vi "RDAOutcouterByMachine.vi"(7 "Machine":string="QAMT08", 8 "error in (no error) 2":errorcluster, 9 "report in":refnum<class "NI_report.lvclass">, 10 "error in (no error)":errorcluster, 11 "connection reference":T1) -> (0 "error in (no error) 3":errorcluster, 1 "report in 2":refnum<class "NI_report.lvclass">, 2 "error out":errorcluster, 3 "connection reference 2":T1)   [LabVIEW 2012]
uses:
  <vilib>/addons/database/Connection.llb/Conn ObjectReference.ctl
  <vilib>/Utility/NIReport.llb/NI_report.lvclass
  <vilib>/addons/database/Auxilliary.llb/DB Tools Cursor Type.ctl
  <vilib>/addons/database/Connection.llb/Conn Execute.vi
  <vilib>/addons/database/Recordset.llb/Rec Fetch Recordset Data (R).vi
  <vilib>/addons/database/Recordset.llb/Rec Destroy - Connection.vi
  <vilib>/addons/database/_DB Variant To Data/Database Variant To Data.xnode
  <vilib>/Utility/NIReport.llb/Excel/NI_Excel.lvclass
  <vilib>/addons/database/NI_Database_API.lvlib
panel:
  out "concatenated string":string
  in  "?":cluster{"start row":i32, "start column":i32}
  in  "?":cluster{"start row":i32, "start column":i32}
  in  "?":cluster{"start row":i32, "start column":i32}
  in  "?":cluster{"start row":i32, "start column":i32}
  in  "?":cluster{"start row":i32, "start column":i32}
  in  "?":cluster{"start row":i32, "start column":i32}
  in  "?":cluster{"start row":i32, "start column":i32}
  in  "?":cluster{"start row":i32, "start column":i32}
  in  "?":cluster{"start row":i32, "start column":i32}
  in  "?":cluster{"start row":i32, "start column":i32}
  in  "?":cluster{"start row":i32, "start column":i32}
  in  "?":cluster{"start row":i32, "start column":i32}
  in  "?":cluster{"start row":i32, "start column":i32}
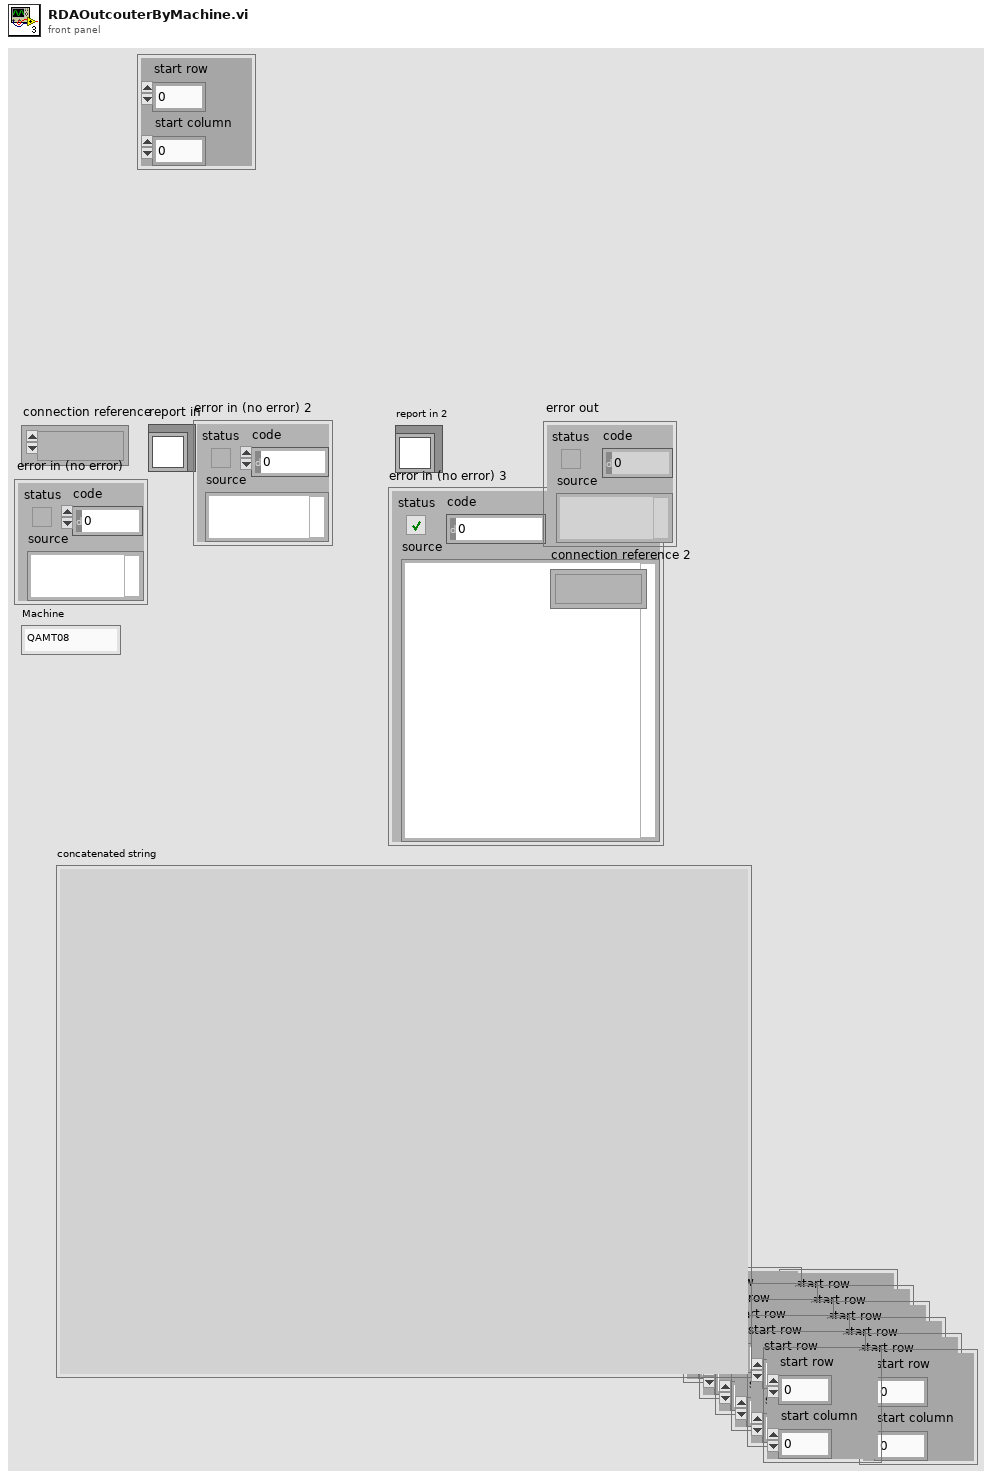
[diagram p1: front panel]
types:
  T1 = typedef "NI_Database_API.lvlib/Conn ObjectReference.ctl" = refnum<k1>
  T2 = typedef "NI_Database_API.lvlib/DB Tools Cursor Type.ctl" = enum16{"forward-only", "keyset", "dynamic", "static"}
  T3 = typedef "NI_Database_API.lvlib/Rec ObjectReference.ctl" = refnum<k1>
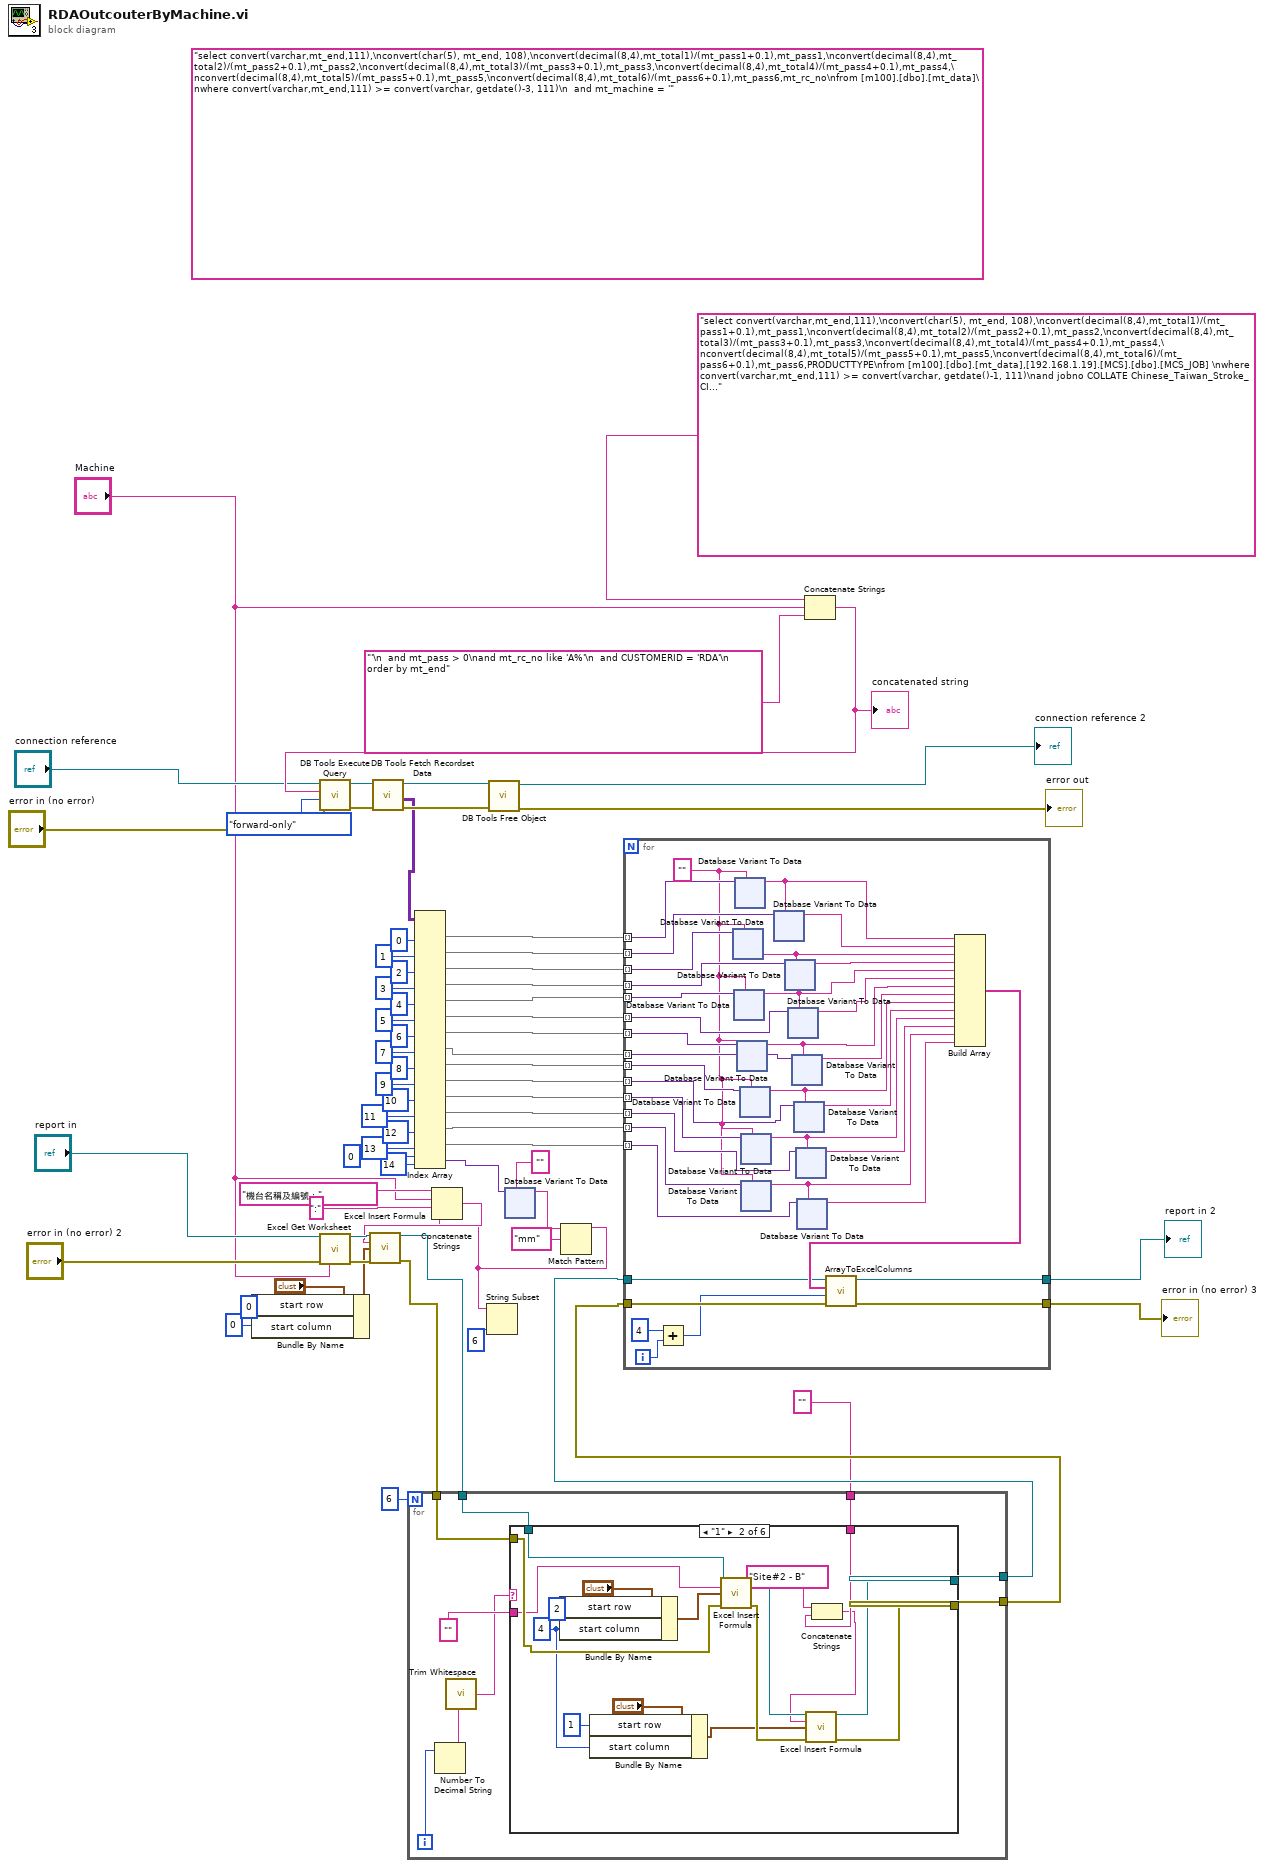
[diagram p0: block diagram]
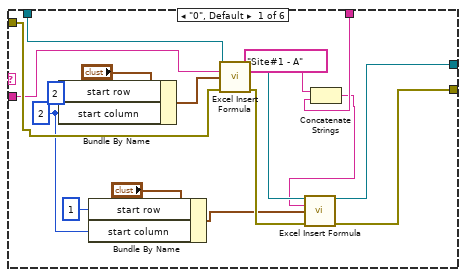
[diagram p2: hidden frame]
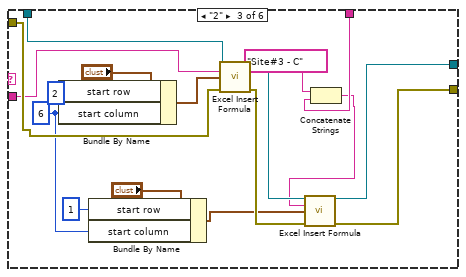
[diagram p3: hidden frame]
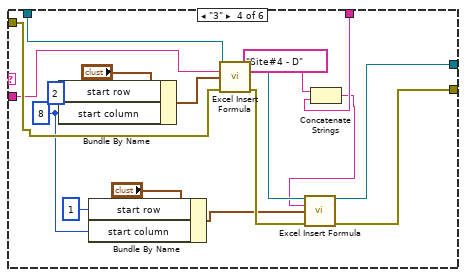
[diagram p4: hidden frame]
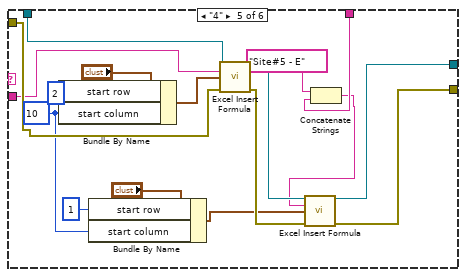
[diagram p5: hidden frame]
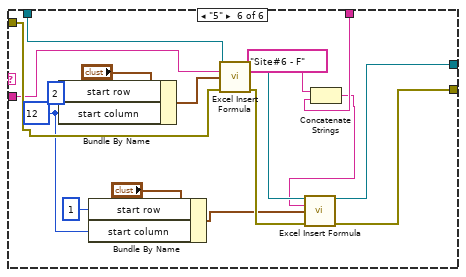
[diagram p6: hidden frame]
diagram:
  (unwired) "select convert(varchar,mt_end,111),\nconvert(char(5), mt_end, 108),\nconvert(decimal(8,4),mt_total1)/(mt_pass1+0.1),mt_pass1,\nconvert(decimal(8,4),mt_total2)/(mt_pass2+0.1),mt_pass2,\nconvert(decimal(8,4),mt_total3)/(mt_pass3+0.1),mt_pass3,\nconvert(decimal(8,4),mt_total4)/(mt_pass4+0.1),mt_pass4,\nconvert(decimal(8,4),mt_total5)/(mt_pass5+0.1),mt_pass5,\nconvert(decimal(8,4),mt_total6)/(mt_pass6+0.1),mt_pass6,mt_rc_no\nfrom [m100].[dbo].[mt_data]\nwhere convert(varchar,mt_end,111) >= convert(varchar, getdate()-3, 111)\n  and mt_machine = '" ("SQL query")
  n1 = Bundle By Name(cluster="?", "start row"=0, "start column"=0) -> (w28:cluster{"start row":i32, "start column":i32})
  n2 = call <vilib>:"Excel Get Worksheet.vi"("report in"="report in", "error in (no error)"="error in (no error) 2", "name (\"\")"="Machine") -> ("report out"=w33:refnum<class "NI_report.lvclass">, "error out"=w32:errorcluster)  [unwired: 11 in]
  n3 = Concatenate Strings("select convert(varchar,mt_end,111),\nconvert(char(5), mt_end, 108),\nconvert(decimal(8,4),mt_total1)/(mt_pass1+0.1),mt_pass1,\nconvert(decimal(8,4),mt_total2)/(mt_pass2+0.1),mt_pass2,\nconvert(decimal(8,4),mt_total3)/(mt_pass3+0.1),mt_pass3,\nconvert(decimal(8,4),mt_total4)/(mt_pass4+0.1),mt_pass4,\nconvert(decimal(8,4),mt_total5)/(mt_pass5+0.1),mt_pass5,\nconvert(decimal(8,4),mt_total6)/(mt_pass6+0.1),mt_pass6,PRODUCTTYPE\nfrom [m100].[dbo].[mt_data],[192.168.1.19].[MCS].[dbo].[MCS_JOB] \nwhere convert(varchar,mt_end,111) >= convert(varchar, getdate()-1, 111)\nand jobno COLLATE Chinese_Taiwan_Stroke_CI_AS = mt_rc_no\n  and mt_machine = '" ("string"), "Machine", "'\n  and mt_pass > 0\nand mt_rc_no like 'A%'\n  and CUSTOMERID = 'RDA'\n  order by mt_end" ("SQL query")) -> (w34:string)
  "concatenated string" <- w34
  n4 = call-poly <vilib>:"DB Tools Execute Query.vi"("error in (no error)"="error in (no error)", "cursor type"=DB_Tools_Cursor_Type."forward-only", "SQL query"=w34, "connection reference"="connection reference") -> ("error out"=w69:errorcluster, "recordset reference"=w68:T3)  [unwired: 4 in]
  n5 = call-poly <vilib>:"DB Tools Fetch Recordset Data.vi"("error in (no error)"=w69, "recordset reference"=w68) -> ("error out"=w66:errorcluster, "recordset data"=w64:variant[][], "recordset reference out"=w67:T3)  [unwired: 3 in]
  n6 = Index Array(array=w64, index (col) #1=0 ("disabled index (col)"), index (col) #2=1 ("index (col)"), index (col) #3=2 ("index (col)"), index (col) #4=3 ("index (col)"), index (col) #5=4 ("index (col)"), index (col) #6=5 ("index (col)"), index (col) #7=6 ("index (col)"), index (col) #8=7 ("index (col)"), index (col) #9=8 ("index (col)"), index (col) #10=9 ("index (col)"), index (col) #11=10 ("index (col)"), index (col) #12=11 ("index (col)"), index (col) #13=12 ("index (col)"), index (col) #14=13 ("index (col)"), index (row) #15=0 ("disabled index (row)"), index (col) #15=14 ("disabled index (col)")) -> (element #1=w61:variant[], element #2=w60:variant[], element #3=w59:variant[], element #4=w48:variant[], element #5=w47:variant[], element #6=w46:variant[], element #7=w45:variant[], element #8=w44:variant[], element #9=w43:variant[], element #10=w42:variant[], element #11=w41:variant[], element #12=w40:variant[], element #13=w37:variant[], element #14=w36:variant[], element #15=w14:variant)  [unwired: 14 in]
  n7 = call-poly <vilib>:"DB Tools Free Object.vi"("error in (no error)"=w66, "recordset reference"=w67) -> ("error out"=→"error out":errorcluster, "connection reference"=→"connection reference 2":T1)  [unwired: 8 in]
  n8 = xnode "Database Variant To Data"("database variant"=w14, "type"="") -> ("data"=w12:string)  [unwired: 1 in, 1 out]
  n9 = Match Pattern(string=w12, regular expression="mm") -> (before substring=w4:string)  [unwired: 1 in, 3 out]
  n10 = Concatenate Strings("機台名稱及編號：" ("formula"), "Machine", ":" ("string"), w4) -> (w27:string)
  n11 = call <vilib>:"Excel Insert Formula.vi"("report in"=w33, "formula"=w27, "start (0, 0)"=w28, "error in (no error)"=w32) -> ("report out"=w10:refnum<class "NI_report.lvclass">, "error out"=w9:errorcluster)  [unwired: 10 in]
  n12 = for {
    N: 6 -> [_]
    tunnel: w10 -> [w78]
    tunnel: w9 -> [w77]
    tunnel: [w76] -> w8
    tunnel: [w75] -> w7
    tunnel: "" -> [w74]
    i -> [w72]
    n13 = Number To Decimal String(number=w72) -> (decimal integer string=w71:string)  [unwired: 1 in]
    n14 = call <vilib>:"Trim Whitespace.vi"("string"=w71) -> ("trimmed string"=w70:string)  [unwired: 1 in]
    n15 = case shown="\"1\"" w70 {
      tunnel: "" -> [w90 w96 w124 w141 w158 w175]
      tunnel: w78 -> [w92 w109 w126 w143 w160 w177]
      tunnel: w77 -> [w91 w108 w125 w142 w159 w176]
      tunnel: [w89 w107 w123 w140 w157 w174] -> w76
      tunnel: [w88 w106 w122 w139 w156 w173] -> w75
      tunnel: w74 -> [w81 w99 w115 w132 w149 w166]
      frame "0", Default {
        w84 = 2 ("start column")
        n16 = Bundle By Name(cluster="?", "start row"=2, "start column"=w84) -> (w93:cluster{"start row":i32, "start column":i32})
        n17 = Bundle By Name(cluster="?", "start row"=1, "start column"=w84) -> (w83:cluster{"start row":i32, "start column":i32})
        n18 = call <vilib>:"Excel Insert Formula.vi"("report in"=w92, "formula"=w90, "start (0, 0)"=w93, "error in (no error)"=w91) -> ("report out"=w80:refnum<class "NI_report.lvclass">, "error out"=w87:errorcluster)  [unwired: 10 in]
        n19 = Concatenate Strings("Site#1 - A" ("string"), w81) -> (w79:string)
        n20 = call <vilib>:"Excel Insert Formula.vi"("report in"=w80, "formula"=w79, "start (0, 0)"=w83, "error in (no error)"=w87) -> ("report out"=w89:refnum<class "NI_report.lvclass">, "error out"=w88:errorcluster)  [unwired: 10 in]
      }
      frame "1" {
        w102 = 4 ("start column")
        n21 = Bundle By Name(cluster="?", "start row"=2, "start column"=w102) -> (w110:cluster{"start row":i32, "start column":i32})
        n22 = Bundle By Name(cluster="?", "start row"=1, "start column"=w102) -> (w101:cluster{"start row":i32, "start column":i32})
        n23 = call <vilib>:"Excel Insert Formula.vi"("report in"=w109, "formula"=w96, "start (0, 0)"=w110, "error in (no error)"=w108) -> ("report out"=w98:refnum<class "NI_report.lvclass">, "error out"=w105:errorcluster)  [unwired: 10 in]
        n24 = Concatenate Strings("Site#2 - B" ("string"), w99) -> (w97:string)
        n25 = call <vilib>:"Excel Insert Formula.vi"("report in"=w98, "formula"=w97, "start (0, 0)"=w101, "error in (no error)"=w105) -> ("report out"=w107:refnum<class "NI_report.lvclass">, "error out"=w106:errorcluster)  [unwired: 10 in]
      }
      frame "2" {
        w118 = 6 ("start column")
        n26 = Bundle By Name(cluster="?", "start row"=2, "start column"=w118) -> (w127:cluster{"start row":i32, "start column":i32})
        n27 = Bundle By Name(cluster="?", "start row"=1, "start column"=w118) -> (w117:cluster{"start row":i32, "start column":i32})
        n28 = call <vilib>:"Excel Insert Formula.vi"("report in"=w126, "formula"=w124, "start (0, 0)"=w127, "error in (no error)"=w125) -> ("report out"=w114:refnum<class "NI_report.lvclass">, "error out"=w121:errorcluster)  [unwired: 10 in]
        n29 = Concatenate Strings("Site#3 - C" ("string"), w115) -> (w113:string)
        n30 = call <vilib>:"Excel Insert Formula.vi"("report in"=w114, "formula"=w113, "start (0, 0)"=w117, "error in (no error)"=w121) -> ("report out"=w123:refnum<class "NI_report.lvclass">, "error out"=w122:errorcluster)  [unwired: 10 in]
      }
      frame "3" {
        w135 = 8 ("start column")
        n31 = Bundle By Name(cluster="?", "start row"=2, "start column"=w135) -> (w144:cluster{"start row":i32, "start column":i32})
        n32 = Bundle By Name(cluster="?", "start row"=1, "start column"=w135) -> (w134:cluster{"start row":i32, "start column":i32})
        n33 = call <vilib>:"Excel Insert Formula.vi"("report in"=w143, "formula"=w141, "start (0, 0)"=w144, "error in (no error)"=w142) -> ("report out"=w131:refnum<class "NI_report.lvclass">, "error out"=w138:errorcluster)  [unwired: 10 in]
        n34 = Concatenate Strings("Site#4 - D" ("string"), w132) -> (w130:string)
        n35 = call <vilib>:"Excel Insert Formula.vi"("report in"=w131, "formula"=w130, "start (0, 0)"=w134, "error in (no error)"=w138) -> ("report out"=w140:refnum<class "NI_report.lvclass">, "error out"=w139:errorcluster)  [unwired: 10 in]
      }
      frame "4" {
        w152 = 10 ("start column")
        n36 = Bundle By Name(cluster="?", "start row"=2, "start column"=w152) -> (w161:cluster{"start row":i32, "start column":i32})
        n37 = Bundle By Name(cluster="?", "start row"=1, "start column"=w152) -> (w151:cluster{"start row":i32, "start column":i32})
        n38 = call <vilib>:"Excel Insert Formula.vi"("report in"=w160, "formula"=w158, "start (0, 0)"=w161, "error in (no error)"=w159) -> ("report out"=w148:refnum<class "NI_report.lvclass">, "error out"=w155:errorcluster)  [unwired: 10 in]
        n39 = Concatenate Strings("Site#5 - E" ("string"), w149) -> (w147:string)
        n40 = call <vilib>:"Excel Insert Formula.vi"("report in"=w148, "formula"=w147, "start (0, 0)"=w151, "error in (no error)"=w155) -> ("report out"=w157:refnum<class "NI_report.lvclass">, "error out"=w156:errorcluster)  [unwired: 10 in]
      }
      frame "5" {
        w169 = 12 ("start column")
        n41 = Bundle By Name(cluster="?", "start row"=2, "start column"=w169) -> (w178:cluster{"start row":i32, "start column":i32})
        n42 = Bundle By Name(cluster="?", "start row"=1, "start column"=w169) -> (w168:cluster{"start row":i32, "start column":i32})
        n43 = call <vilib>:"Excel Insert Formula.vi"("report in"=w177, "formula"=w175, "start (0, 0)"=w178, "error in (no error)"=w176) -> ("report out"=w165:refnum<class "NI_report.lvclass">, "error out"=w172:errorcluster)  [unwired: 10 in]
        n44 = Concatenate Strings("Site#6 - F" ("string"), w166) -> (w164:string)
        n45 = call <vilib>:"Excel Insert Formula.vi"("report in"=w165, "formula"=w164, "start (0, 0)"=w168, "error in (no error)"=w172) -> ("report out"=w174:refnum<class "NI_report.lvclass">, "error out"=w173:errorcluster)  [unwired: 10 in]
      }
    }
  }
  n46 = String Subset(string=w4, length (rest)=6 ("length (rest)")) -> ()  [unwired: 1 in, 1 out]
  n47 = for {
    tunnel: w61 -> [w217] mode=indexing
    tunnel: w60 -> [w216] mode=indexing
    tunnel: w59 -> [w215] mode=indexing
    tunnel: w48 -> [w213] mode=indexing
    tunnel: w47 -> [w209] mode=indexing
    tunnel: w46 -> [w207] mode=indexing
    tunnel: w45 -> [w205] mode=indexing
    tunnel: w44 -> [w202] mode=indexing
    tunnel: w43 -> [w201] mode=indexing
    tunnel: w42 -> [w200] mode=indexing
    tunnel: w41 -> [w197] mode=indexing
    tunnel: w40 -> [w196] mode=indexing
    tunnel: w37 -> [w193] mode=indexing
    tunnel: w36 -> [w192] mode=indexing
    tunnel: w8 -> [w187]
    tunnel: w7 -> [w186]
    tunnel: [w182] -> w21
    tunnel: [w181] -> w20
    i -> [w185]
    w189 = ""
    n48 = Add(x=4, y=w185) -> (x+y=w183:i32)
    n49 = xnode "Database Variant To Data"("database variant"=w215, "type"=w189) -> ("data"=w211:string)  [unwired: 1 in, 1 out]
    n50 = xnode "Database Variant To Data"("database variant"=w209, "type"=w189) -> ("data"=w208:string)  [unwired: 1 in, 1 out]
    n51 = xnode "Database Variant To Data"("database variant"=w217, "type"=w189) -> ("data"=w212:string)  [unwired: 1 in, 1 out]
    n52 = xnode "Database Variant To Data"("database variant"=w205, "type"=w189) -> ("data"=w204:string)  [unwired: 1 in, 1 out]
    n53 = xnode "Database Variant To Data"("database variant"=w201, "type"=w189) -> ("data"=w199:string)  [unwired: 1 in, 1 out]
    n54 = xnode "Database Variant To Data"("database variant"=w197, "type"=w189) -> ("data"=w195:string)  [unwired: 1 in, 1 out]
    n55 = xnode "Database Variant To Data"("database variant"=w193, "type"=w189) -> ("data"=w191:string)  [unwired: 1 in, 1 out]
    n56 = xnode "Database Variant To Data"("database variant"=w216, "type"=w212) -> ("data"=w214:string)  [unwired: 1 in, 1 out]
    n57 = xnode "Database Variant To Data"("database variant"=w213, "type"=w211) -> ("data"=w210:string)  [unwired: 1 in, 1 out]
    n58 = xnode "Database Variant To Data"("database variant"=w207, "type"=w208) -> ("data"=w206:string)  [unwired: 1 in, 1 out]
    n59 = xnode "Database Variant To Data"("database variant"=w202, "type"=w204) -> ("data"=w203:string)  [unwired: 1 in, 1 out]
    n60 = xnode "Database Variant To Data"("database variant"=w200, "type"=w199) -> ("data"=w198:string)  [unwired: 1 in, 1 out]
    n61 = xnode "Database Variant To Data"("database variant"=w196, "type"=w195) -> ("data"=w194:string)  [unwired: 1 in, 1 out]
    n62 = xnode "Database Variant To Data"("database variant"=w192, "type"=w191) -> ("data"=w190:string)  [unwired: 1 in, 1 out]
    n63 = Build Array(w212, w214, w211, w210, w208, w206, w204, w203, w199, w198, w195, w194, w191, w190) -> (w188:string[])
    n64 = call "ArrayToExcelColumns.vi"("error in (no error)"=w186, "start row"=w183, "ArrayData"=w188, "report in"=w187) -> ("error in (no error) 2"=w181:errorcluster, "report in 2"=w182:refnum<class "NI_report.lvclass">)  [unwired: 6 in]
  }
  "report in 2" <- w21
  "error in (no error) 3" <- w20
